vi "Read 2D Array From XL.vi"(8 "error in":errorcluster, 9 "Write/Read Cell":T1={"Cell Range"="", "Data 2D"=[], "Select Sheet"="", "1 Data"="", "Data 1D"=[], "Font col"=0, "Bold"=TRUE, "Font Size"=18, "Inside lines"=FALSE}, 10 "Work Sheet":refnum<k7>, 11 "Excel._Workbook":refnum<k7>) -> (0 "error out":errorcluster, 1 "Data From Cells":string[][](array[string]), 2 "Work Sheet":refnum<k7>, 3 "Excel._Workbook":refnum<k7>)   [LabVIEW 2017]
uses:
  controls/read.write.ctl
panel:
  out "Value2":variant
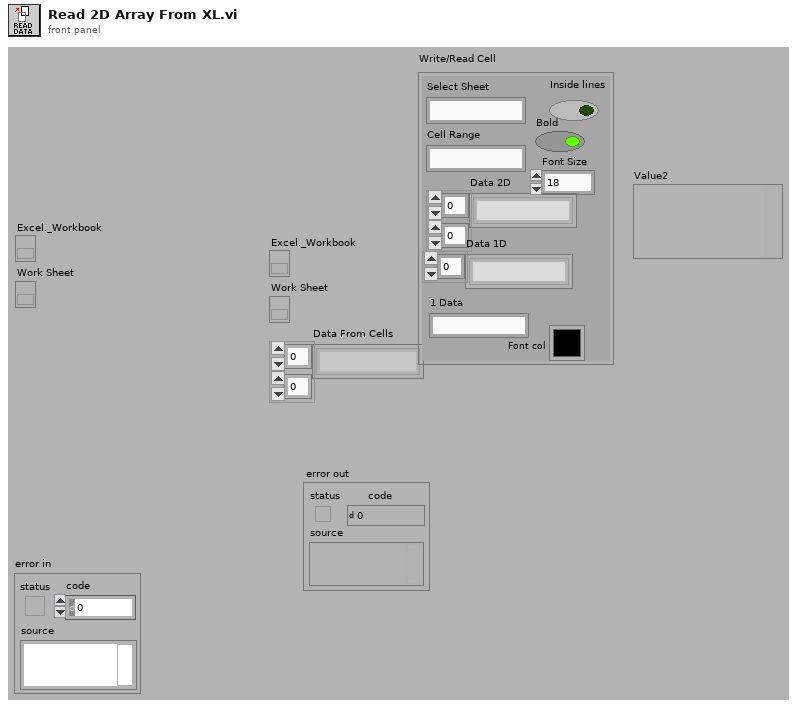
[diagram p1: front panel]
types:
  T1 = typedef "read.write.ctl" = cluster{"Cell Range":string, "Data 2D":string[][], "Select Sheet":string, "1 Data":string, "Data 1D":string[], "Font col":u32, "Bold":bool, "Font Size":i32, "Inside lines":bool}
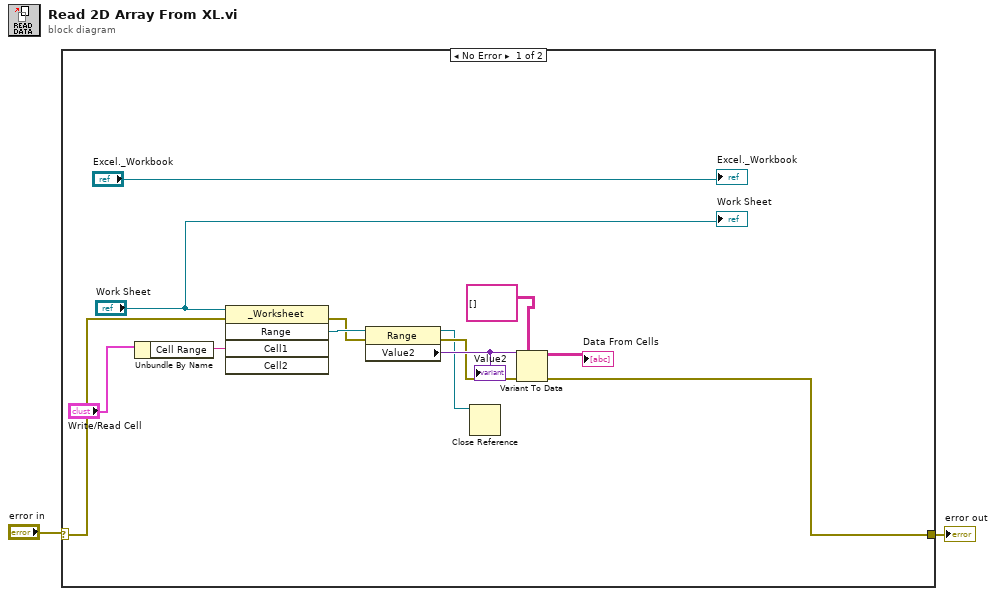
[diagram p0: block diagram]
diagram:
  n1 = case shown="No Error" "error in" {
    selector: "error in" -> [w12 w16]
    tunnel: [w9 w16] -> w1
    frame No Error {
      n2 = Unbundle By Name("Write/Read Cell") -> ("Cell Range"=w5:string)
      n3 = invoke class="_Worksheet" method="Range"(reference="Work Sheet", error in=w12, "Cell1"=w5) -> (error out=w11:errorcluster, "Range"=w14:refnum<k7>)  [unwired: 2 in, 3 out]
      n4 = property class="Range"(reference=w14, error in=w11) -> (reference out=w4:refnum<k7>, error out=w10:errorcluster, "Value2"=w13:variant)
      "Value2" <- w13
      n5 = Close Reference(reference=w4) -> ()  [unwired: 1 in, 1 out]
      n6 = Variant To Data(error in=w10, type=string[][] [], Variant=w13) -> (data=→"Data From Cells":string[][], error out=w9:errorcluster)
      "Work Sheet" <- "Work Sheet"
      "Excel._Workbook" <- "Excel._Workbook"
    }
    frame Error {
    }
  }
  "error out" <- w1
